vi "SSC Digital Get HRAM Settings.vi"(0 "Digital SSC in":T1[](array[typedef]), 11 "error in":errorcluster) -> (3 "Per-Instrument Number of Samples is Finite":bool[](array[boolean]), 4 "Digital SSC out":T1[](array[typedef]), 6 "Per-Instrument Cycles to Acquire":i32[](array[ring]) items=["Failed Cycles"=2303, "All Cycles"=2304], 8 "Per-Instrument Pretrigger Samples":i32[](array[numeric]), 10 "Per-Instrument Buffer Size Per Site":i64[](array[numeric]), 14 "Per-Instrument Max Samples To Acquire Per Site":i32[](array[numeric]), 15 "error out":errorcluster)   [LabVIEW 2019]
doc: "Uses the start label you specify to burst the pattern on the pin(s) and pin group(s) you specify."
uses:
  SSC Digital.ctl
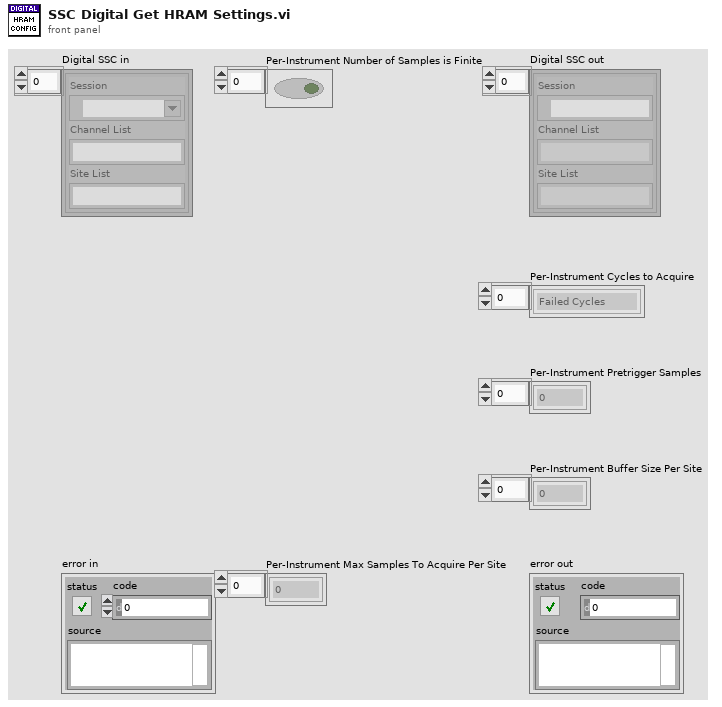
[diagram p1: front panel]
types:
  T1 = typedef "SSC Digital.ctl" = cluster{"Session":refnum<k15>, "Channel List":string, "Site List":string}
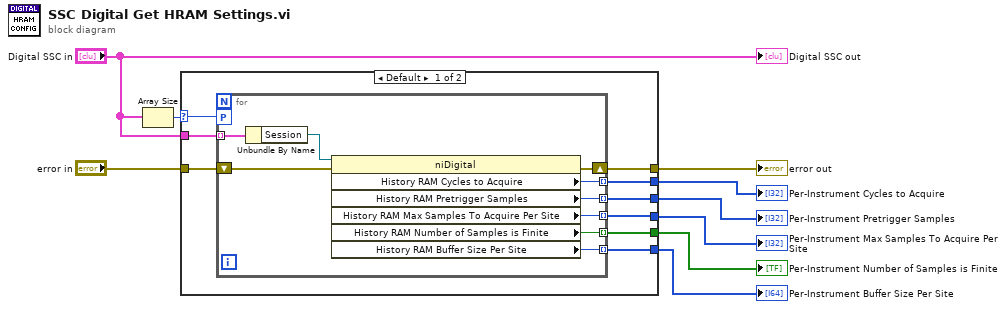
[diagram p0: block diagram]
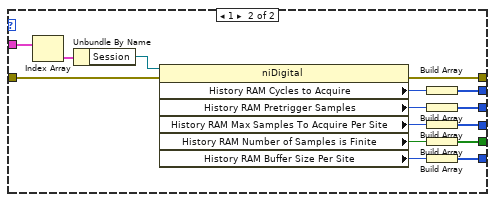
[diagram p2: hidden frame]
diagram:
  n1 = Array Size(array="Digital SSC in") -> (size(s)=w8:i32)
  n2 = case shown="Default" w8 {
    selector: w8 -> [w18 _]
    tunnel: "error in" -> [w16 w41]
    tunnel: "Digital SSC in" -> [w17 w42]
    tunnel: [w15 w40] -> w6
    tunnel: [w14 w28] -> w1
    tunnel: [w13 w29] -> w2
    tunnel: [w12 w30] -> w3
    tunnel: [w11 w31] -> w4
    tunnel: [w10 w32] -> w5
    frame Default {
      n3 = for {
        tunnel: w17 -> [w27] mode=indexing
        workers-P: w18 -> [_]
        shift-right: [w26] -> w15
        shift-left: w16 -> [w24]
        tunnel: [w23] -> w14 mode=indexing
        tunnel: [w22] -> w13 mode=indexing
        tunnel: [w21] -> w12 mode=indexing
        tunnel: [w20] -> w11 mode=indexing
        tunnel: [w19] -> w10 mode=indexing
        n4 = Unbundle By Name(w27) -> ("Session"=w25:refnum<k15>)
        n5 = property class="niDigital"(reference=w25, error in=w24) -> (error out=w26:errorcluster, "History RAM Cycles to Acquire"=w19:i32, "History RAM Pretrigger Samples"=w20:i32, "History RAM Max Samples To Acquire Per Site"=w21:i32, "History RAM Number of Samples is Finite"=w22:bool, "History RAM Buffer Size Per Site"=w23:i64)  [unwired: 1 out]
      }
    }
    frame 1 {
      n6 = Index Array(array=w42) -> (element=w38:T1)  [unwired: 1 in]
      n7 = Unbundle By Name(w38) -> ("Session"=w39:refnum<k15>)
      n8 = property class="niDigital"(reference=w39, error in=w41) -> (error out=w40:errorcluster, "History RAM Cycles to Acquire"=w37:i32, "History RAM Pretrigger Samples"=w36:i32, "History RAM Max Samples To Acquire Per Site"=w35:i32, "History RAM Number of Samples is Finite"=w34:bool, "History RAM Buffer Size Per Site"=w33:i64)  [unwired: 1 out]
      n9 = Build Array(w37) -> (w32:i32[])
      n10 = Build Array(w36) -> (w31:i32[])
      n11 = Build Array(w35) -> (w30:i32[])
      n12 = Build Array(w34) -> (w29:bool[])
      n13 = Build Array(w33) -> (w28:i64[])
    }
  }
  "error out" <- w6
  "Per-Instrument Cycles to Acquire" <- w5
  "Per-Instrument Pretrigger Samples" <- w4
  "Per-Instrument Max Samples To Acquire Per Site" <- w3
  "Per-Instrument Number of Samples is Finite" <- w2
  "Per-Instrument Buffer Size Per Site" <- w1
  "Digital SSC out" <- "Digital SSC in"
